vi "Remove Helper Extension.vi"(11 "Filename":string) -> (3 "Filename without Helper Extension":string)   [LabVIEW 2020, in "VI Properties Editor.lvlib" / "Project Tree Map.lvclass"]
uses:
  Project Tree Map.lvclass
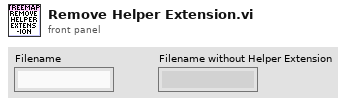
[diagram p1: front panel]
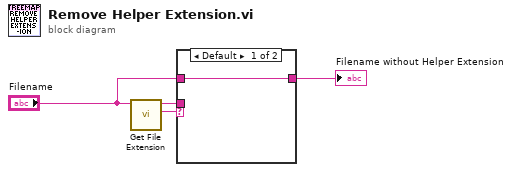
[diagram p0: block diagram]
diagram:
  n1 = call "Get File Extension.vi"("Filename"="Filename") -> ("Lowercase Extension"=w4:string, "Filename without Extension"=w3:string)  [unwired: 9 in]
  n2 = case shown="Default" w4 {
    selector: w4 -> [_ w6]
    tunnel: w3 -> [_ _]
    tunnel: "Filename" -> [w5 _]
    tunnel: [w5 w6] -> w1
    frame Default {
    }
    frame "target", "virtual" {
    }
  }
  "Filename without Helper Extension" <- w1
